vi "Set Output Switch Direction.vi"(8 "error in (no error)":errorcluster, 10 "After delay":bool, 11 "RP Instrument in":refnum<class "RP Instrument.lvclass">) -> (0 "error out":errorcluster, 3 "RP Instrument out":refnum<class "RP Instrument.lvclass">)   [LabVIEW 2019, in "RP Instrument.lvclass"]
uses:
  RP Instrument.lvclass
  RP Command.ctl
  RP Instrument.lvclass/RP Instrument.ctl
  RP Communicator/RP Communicator.lvclass
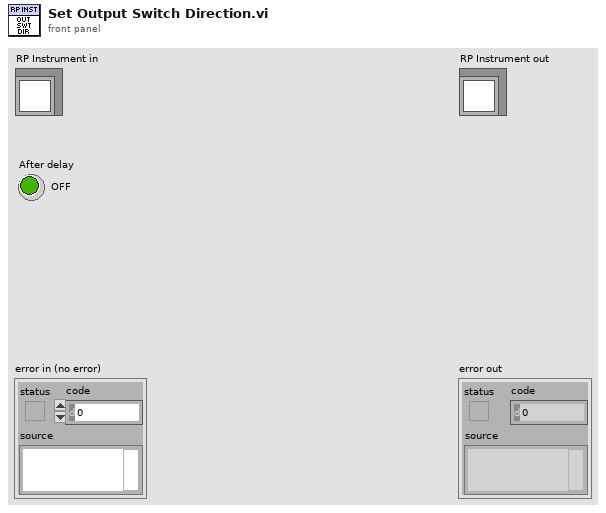
[diagram p1: front panel]
types:
  T1 = typedef "RP Command.ctl" = enum16{"Reset", "Read IDN", "Stop server", "Get status", "Get temperature", "Connect client", "Arm", "Software trigger", "Get whole buffer", "Get chunk", "System call", "Get config", "Set config", "Recieve data", "Recieve Calibartion", "Transmit data"}
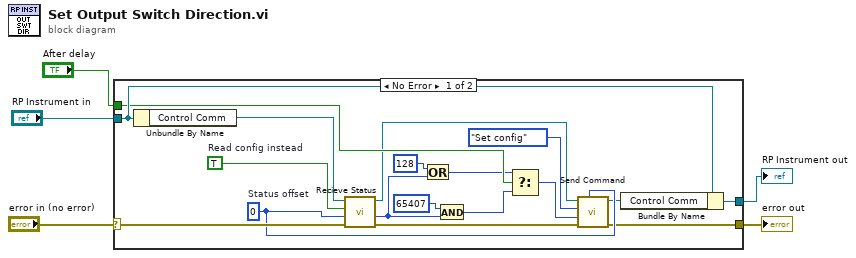
[diagram p0: block diagram]
diagram:
  n1 = case shown="No Error" "error in (no error)" {
    selector: "error in (no error)" -> [w20 w25]
    tunnel: [w8 w25] -> w4
    tunnel: [w7 w24] -> w2
    tunnel: "RP Instrument in" -> [w23 w24]
    tunnel: "After delay" -> [w19 _]
    frame No Error {
      w11 = u64 0  # Status offset
      w21 = TRUE  # Read config instead
      n2 = Unbundle By Name(w23) -> ("Control Comm"=w22:refnum<class "RP Communicator.lvclass">)
      n3 = call-dynamic "Recieve Status.vi"("error in (no error)"=w20, "Status offset"=w11, "Read config instead"=w21, "RP Communicator in"=w22) -> ("error out"=w9:errorcluster, "Status response"=w15:u32, "RP Communicator out"=w13:refnum<class "RP Communicator.lvclass">)  [unwired: 5 in]
      n4 = Or(x=u32 128, y=w15) -> (x .or. y?=w14:u32)
      n5 = And(x=u32 65407, y=w15) -> (x .and. y?=w17:u32)
      n6 = Select(t=w14, s=w19, f=w17) -> (s? t:f=w10:u32)
      n7 = call-dynamic "Send Command.vi"("Config offset"=w11, "error in (no error)"=w9, "Command payload"=w10, "Command number"=RP_Command."Set config", "RP Communicator in"=w13) -> ("error out"=w8:errorcluster, "RP Communicator out"=w6:refnum<class "RP Communicator.lvclass">)  [unwired: 5 in]
      n8 = Bundle By Name(cluster=w23, "Control Comm"=w6) -> (w7:refnum<class "RP Instrument.lvclass">)
    }
    frame Error {
    }
  }
  "error out" <- w4
  "RP Instrument out" <- w2
